vi "1L17_theC-T-en-Volts.vi"(5 "Temperature Units":u16(ring) caption="Unités de température" items=["Celsius", "Fahrenheit", "Kelvin", "Rankine"], 6 "ThermocoupleType":u16(ring)=2 caption="TypeThermocouple" items=["B", "E", "J", "K", "R", "S", "T", "N"], 7 "Temperature":sgl caption="Température" format="%0.6f") -> (3 "Thermocouple Voltage":sgl caption="Tension du thermocouple" format="%0.6f")   [LabVIEW 2010, in "lv_01.lvlib"]
doc: "Convertit une température en tension de thermocouple.\n\nNational Instruments a choisi des expressions polynomiales de thermocouple qui ne sont valides que pour des gammes de températures spécifiques (indiquées sur le diagramme du VI). Ces polynômes proviennent des tables NIST Monograph 175.\n\nPour utiliser une autre formule de conversion, vous pouvez éditer ce VI et entrer votre propre formule dans la boîte de calcul appropriée."
uses:
  lv_01.lvlib
panel:
  # "Convertit une température en une tension de thermocouple."
  # "National Instruments a sélectionné des expressions polynomiale de thermocouple qui ne sont valides que pour des gammes de températures particulières (données dans le diagramme du VI)  Ces polynômes proviennent des tables NIST Monograph 175.\n\nPour utiliser une autre formule de conversion, vous pouvez éditer ce VI et entrer votre propre formule dans la boîte de calcul appropriée."
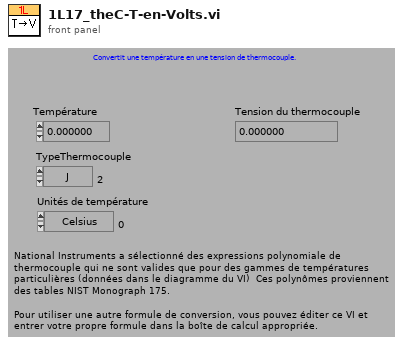
[diagram p1: front panel]
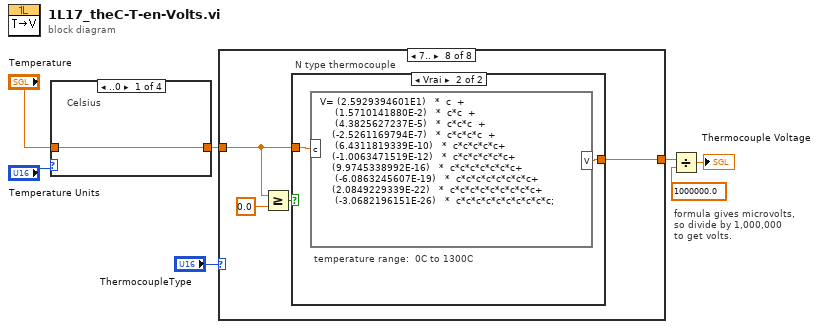
[diagram p0: block diagram]
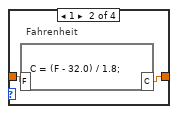
[diagram p2: hidden frame]
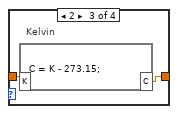
[diagram p3: hidden frame]
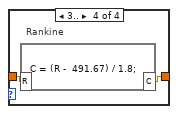
[diagram p4: hidden frame]
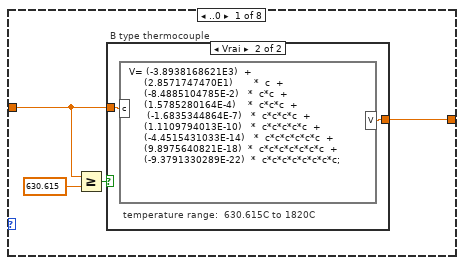
[diagram p5: hidden frame]
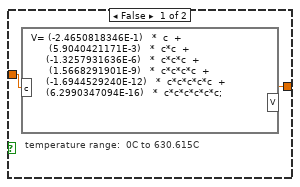
[diagram p6: hidden frame]
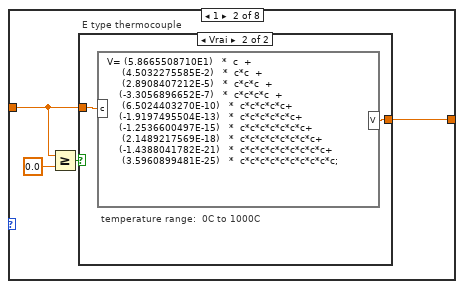
[diagram p7: hidden frame]
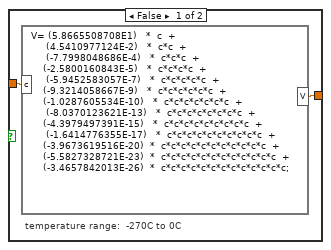
[diagram p8: hidden frame]
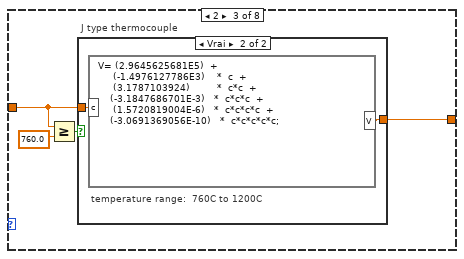
[diagram p9: hidden frame]
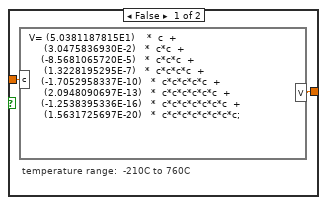
[diagram p10: hidden frame]
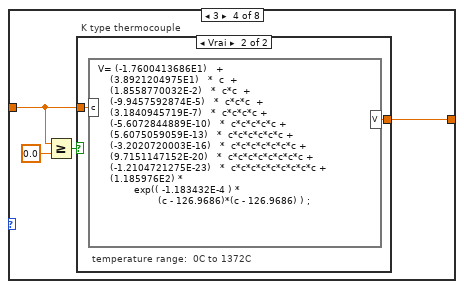
[diagram p11: hidden frame]
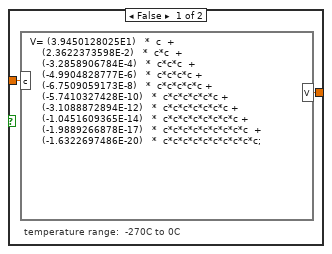
[diagram p12: hidden frame]
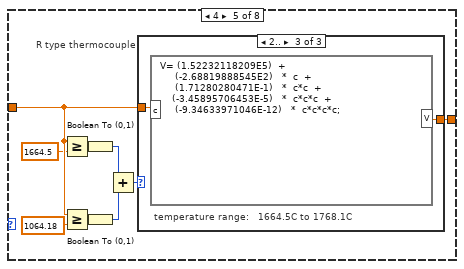
[diagram p13: hidden frame]
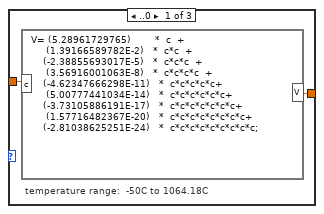
[diagram p14: hidden frame]
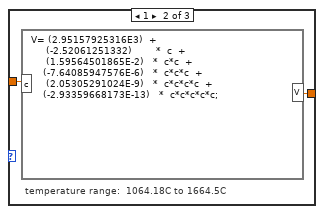
[diagram p15: hidden frame]
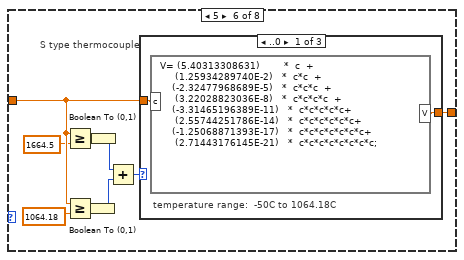
[diagram p16: hidden frame]
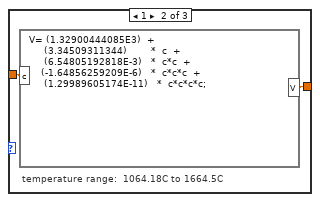
[diagram p17: hidden frame]
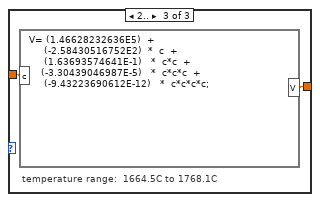
[diagram p18: hidden frame]
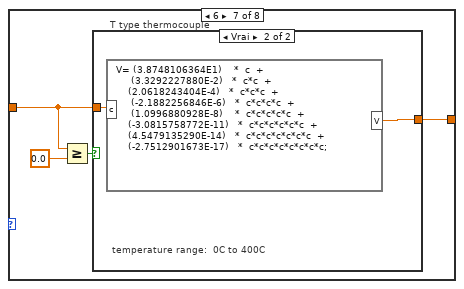
[diagram p19: hidden frame]
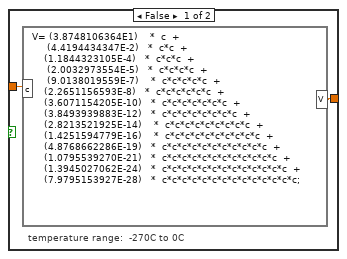
[diagram p20: hidden frame]
diagram:
  # "formula gives microvolts,\nso divide by 1,000,000\nto get volts."
  n1 = case shown="..0" "Temperature Units" {
    tunnel: "Temperature" -> [w8 w10 w12 w14]
    tunnel: [w8 w9 w11 w13] -> w6
    frame ..0 {
      # "Celsius"
    }
    frame 1 {
      # "Fahrenheit"
      n2 = formula code="C = (F - 32.0) / 1.8;"("F"=w10) -> ("C"=w9:dbl)
    }
    frame 2 {
      # "Kelvin"
      n3 = formula code="C = K - 273.15;"("K"=w12) -> ("C"=w11:dbl)
    }
    frame 3.. {
      # "Rankine"
      n4 = formula code="C = (R -  491.67) / 1.8;"("R"=w14) -> ("C"=w13:dbl)
    }
  }
  n5 = case shown="7.." "ThermocoupleType" {
    tunnel: [w15 w26 w34 w42 w55 w70 w80 w85] -> w3
    tunnel: w6 -> [w17 w24 w32 w40 w53 w68 w78 w86]
    frame ..0 {
      # "B type thermocouple"
      n6 = Greater Or Equal?(x=w17, y=630.615) -> (x >= y?=w18:bool)
      n7 = case shown="Vrai" w18 {
        tunnel: w17 -> [w19 w22]
        tunnel: [w20 w21] -> w15
        frame False {
          # "temperature range:  0C to 630.615C"
          n8 = formula code="V= (-2.4650818346E-1)   *  c  +\n      (5.9040421171E-3)   *  c*c  +\n     (-1.3257931636E-6)   *  c*c*c  +\n      (1.5668291901E-9)   *  c*c*c*c  +\n     (-1.6944529240E-12)   *  c*c*c*c*c  +\n     (6.2990347094E-16)   *  c*c*c*c*c*c;"("c"=w19) -> ("V"=w20:dbl)
        }
        frame True {
          # "temperature range:  630.615C to 1820C"
          n9 = formula code="V= (-3.8938168621E3)  +\n     (2.8571747470E1)       *  c  +\n     (-8.4885104785E-2)   *  c*c  +\n     (1.5785280164E-4)    *  c*c*c  +\n      (-1.6835344864E-7)   *  c*c*c*c  +\n     (1.1109794013E-10)   *  c*c*c*c*c  +\n     (-4.4515431033E-14)   *  c*c*c*c*c*c  +\n     (9.8975640821E-18)  *  c*c*c*c*c*c*c  +\n     (-9.3791330289E-22)  *  c*c*c*c*c*c*c*c;"("c"=w22) -> ("V"=w21:dbl)
        }
      }
    }
    frame 1 {
      # "E type thermocouple"
      n10 = Greater Or Equal?(x=w24, y=0.0) -> (x >= y?=w25:bool)
      n11 = case shown="Vrai" w25 {
        tunnel: w24 -> [w28 w30]
        tunnel: [w27 w29] -> w26
        frame False {
          # "temperature range:  -270C to 0C"
          n12 = formula code="V= (5.8665508708E1)   *  c  +\n     (4.5410977124E-2)   *  c*c  +\n     (-7.7998048686E-4)   *  c*c*c  +\n    (-2.5800160843E-5)   *  c*c*c*c  +\n     (-5.9452583057E-7)   *  c*c*c*c*c  +\n    (-9.3214058667E-9)   *  c*c*c*c*c*c  +\n    (-1.0287605534E-10)   *  c*c*c*c*c*c*c  +\n     (-8.0370123621E-13)   *  c*c*c*c*c*c*c*c  +\n    (-4.3979497391E-15)   *  c*c*c*c*c*c*c*c*c  +\n     (-1.6414776355E-17)   *  c*c*c*c*c*c*c*c*c*c  +\n    (-3.9673619516E-20)  *  c*c*c*c*c*c*c*c*c*c*c  +\n    (-5.5827328721E-23)  *  c*c*c*c*c*c*c*c*c*c*c*c  +\n    (-3.4657842013E-26)  *  c*c*c*c*c*c*c*c*c*c*c*c*c;"("c"=w28) -> ("V"=w27:dbl)
        }
        frame True {
          # "temperature range:  0C to 1000C"
          n13 = formula code="V= (5.8665508710E1)   *  c  +\n     (4.5032275585E-2)   *  c*c  +\n     (2.8908407212E-5)   *  c*c*c  +\n    (-3.3056896652E-7)   *  c*c*c*c  +\n     (6.5024403270E-10)   *  c*c*c*c*c+\n    (-1.9197495504E-13)   *  c*c*c*c*c*c+\n    (-1.2536600497E-15)   *  c*c*c*c*c*c*c+\n     (2.1489217569E-18)   *  c*c*c*c*c*c*c*c+\n    (-1.4388041782E-21)   *  c*c*c*c*c*c*c*c*c+\n     (3.5960899481E-25)   *  c*c*c*c*c*c*c*c*c*c;"("c"=w30) -> ("V"=w29:dbl)
        }
      }
    }
    frame 2 {
      # "J type thermocouple"
      n14 = Greater Or Equal?(x=w32, y=760.0) -> (x >= y?=w33:bool)
      n15 = case shown="Vrai" w33 {
        tunnel: [w36 w38] -> w34
        tunnel: w32 -> [w35 w37]
        frame False {
          # "temperature range:  -210C to 760C"
          n16 = formula code="V= (5.0381187815E1)    *  c  +\n     (3.0475836930E-2)   *  c*c  +\n    (-8.5681065720E-5)   *  c*c*c  +\n     (1.3228195295E-7)   *  c*c*c*c  +\n    (-1.7052958337E-10)   *  c*c*c*c*c  +\n     (2.0948090697E-13)   *  c*c*c*c*c*c  +\n    (-1.2538395336E-16)   *  c*c*c*c*c*c*c  +\n     (1.5631725697E-20)   *  c*c*c*c*c*c*c*c;"("c"=w35) -> ("V"=w36:dbl)
        }
        frame True {
          # "temperature range:  760C to 1200C"
          n17 = formula code="V= (2.9645625681E5)  +\n     (-1.4976127786E3)    *  c  +\n     (3.1787103924)         *  c*c  +\n    (-3.1847686701E-3)   *  c*c*c  +\n     (1.5720819004E-6)   *  c*c*c*c  +\n    (-3.0691369056E-10)   *  c*c*c*c*c;"("c"=w37) -> ("V"=w38:dbl)
        }
      }
    }
    frame 3 {
      # "K type thermocouple"
      n18 = Greater Or Equal?(x=w40, y=0.0) -> (x >= y?=w41:bool)
      n19 = case shown="Vrai" w41 {
        tunnel: w40 -> [w44 w46]
        tunnel: [w43 w45] -> w42
        frame False {
          # "temperature range:  -270C to 0C"
          n20 = formula code="V= (3.9450128025E1)   *  c  +\n    (2.3622373598E-2)   *  c*c  +\n    (-3.2858906784E-4)   *  c*c*c  +\n    (-4.9904828777E-6)   *  c*c*c*c +\n    (-6.7509059173E-8)   *  c*c*c*c*c +\n    (-5.7410327428E-10)   *  c*c*c*c*c*c +\n    (-3.1088872894E-12)   *  c*c*c*c*c*c*c +\n    (-1.0451609365E-14)   *  c*c*c*c*c*c*c*c +\n    (-1.9889266878E-17)   *  c*c*c*c*c*c*c*c*c  +\n    (-1.6322697486E-20)   *  c*c*c*c*c*c*c*c*c*c;"("c"=w44) -> ("V"=w43:dbl)
        }
        frame True {
          # "temperature range:  0C to 1372C"
          n21 = formula code="V= (-1.7600413686E1)   +\n    (3.8921204975E1)   *  c  +\n    (1.8558770032E-2)   *  c*c  +\n    (-9.9457592874E-5)   *  c*c*c  +\n    (3.1840945719E-7)   *  c*c*c*c +\n    (-5.6072844889E-10)   *  c*c*c*c*c +\n    (5.6075059059E-13)   *  c*c*c*c*c*c +\n    (-3.2020720003E-16)   *  c*c*c*c*c*c*c +\n    (9.7151147152E-20)   *  c*c*c*c*c*c*c*c +\n    (-1.2104721275E-23)   *  c*c*c*c*c*c*c*c*c +\n    (1.185976E2) * \n            exp(( -1.183432E-4 ) * \n                    (c - 126.9686)*(c - 126.9686) ) ;"("c"=w46) -> ("V"=w45:dbl)
        }
      }
    }
    frame 4 {
      # "R type thermocouple"
      n22 = Greater Or Equal?(x=w53, y=1664.5) -> (x >= y?=w50:bool)
      n23 = Greater Or Equal?(x=w53, y=1064.18) -> (x >= y?=w49:bool)
      n24 = Boolean To (0,1)(Boolean=w50) -> (0, 1=w47:i16)
      n25 = Boolean To (0,1)(Boolean=w49) -> (0, 1=w48:i16)
      n26 = Add(x=w47, y=w48) -> (x+y=w54:i16)
      n27 = case shown="2.." w54 {
        tunnel: w53 -> [w57 w59 w61]
        tunnel: [w56 w58 w60] -> w55
        frame ..0 {
          # "temperature range:  -50C to 1064.18C"
          n28 = formula code="V= (5.28961729765)        *  c  +\n     (1.39166589782E-2)   *  c*c  +\n    (-2.38855693017E-5)   *  c*c*c  +\n     (3.56916001063E-8)   *  c*c*c*c  +\n    (-4.62347666298E-11)   *  c*c*c*c*c+\n     (5.00777441034E-14)   *  c*c*c*c*c*c+\n    (-3.73105886191E-17)   *  c*c*c*c*c*c*c+\n     (1.57716482367E-20)   *  c*c*c*c*c*c*c*c+\n    (-2.81038625251E-24)   *  c*c*c*c*c*c*c*c*c;"("c"=w57) -> ("V"=w56:dbl)
        }
        frame 1 {
          # "temperature range:  1064.18C to 1664.5C"
          n29 = formula code="V= (2.95157925316E3)  +\n     (-2.52061251332)        *  c  +\n     (1.59564501865E-2)   *  c*c  +\n    (-7.64085947576E-6)   *  c*c*c  +\n     (2.05305291024E-9)   *  c*c*c*c  +\n    (-2.93359668173E-13)   *  c*c*c*c*c;"("c"=w59) -> ("V"=w58:dbl)
        }
        frame 2.. {
          # "temperature range:   1664.5C to 1768.1C"
          n30 = formula code="V= (1.52232118209E5)  +\n     (-2.68819888545E2)   *  c  +\n     (1.71280280471E-1)   *  c*c  +\n    (-3.45895706453E-5)   *  c*c*c  +\n     (-9.34633971046E-12)   *  c*c*c*c;"("c"=w61) -> ("V"=w60:dbl)
        }
      }
    }
    frame 5 {
      # "S type thermocouple"
      n31 = Greater Or Equal?(x=w68, y=1664.5) -> (x >= y?=w65:bool)
      n32 = Greater Or Equal?(x=w68, y=1064.18) -> (x >= y?=w64:bool)
      n33 = Boolean To (0,1)(Boolean=w64) -> (0, 1=w63:i16)
      n34 = Boolean To (0,1)(Boolean=w65) -> (0, 1=w62:i16)
      n35 = Add(x=w62, y=w63) -> (x+y=w69:i16)
      n36 = case shown="..0" w69 {
        tunnel: w68 -> [w72 w74 w76]
        tunnel: [w71 w73 w75] -> w70
        frame ..0 {
          # "temperature range:  -50C to 1064.18C"
          n37 = formula code="V= (5.40313308631)        *  c  +\n     (1.25934289740E-2)   *  c*c  +\n    (-2.32477968689E-5)   *  c*c*c  +\n     (3.22028823036E-8)   *  c*c*c*c  +\n    (-3.31465196389E-11)   *  c*c*c*c*c+\n     (2.55744251786E-14)   *  c*c*c*c*c*c+\n    (-1.25068871393E-17)   *  c*c*c*c*c*c*c+\n     (2.71443176145E-21)   *  c*c*c*c*c*c*c*c;"("c"=w72) -> ("V"=w71:dbl)
        }
        frame 1 {
          # "temperature range:  1064.18C to 1664.5C"
          n38 = formula code="V= (1.32900444085E3)  +\n     (3.34509311344)        *  c  +\n     (6.54805192818E-3)   *  c*c  +\n    (-1.64856259209E-6)   *  c*c*c  +\n     (1.29989605174E-11)   *  c*c*c*c;"("c"=w74) -> ("V"=w73:dbl)
        }
        frame 2.. {
          # "temperature range:  1664.5C to 1768.1C"
          n39 = formula code="V= (1.46628232636E5)  +\n     (-2.58430516752E2)  *  c  +\n     (1.63693574641E-1)   *  c*c  +\n    (-3.30439046987E-5)   *  c*c*c  +\n     (-9.43223690612E-12)   *  c*c*c*c;"("c"=w76) -> ("V"=w75:dbl)
        }
      }
    }
    frame 6 {
      # "T type thermocouple"
      n40 = Greater Or Equal?(x=w78, y=0.0) -> (x >= y?=w79:bool)
      n41 = case shown="Vrai" w79 {
        tunnel: w78 -> [w82 w84]
        tunnel: [w81 w83] -> w80
        frame False {
          # "temperature range:  -270C to 0C"
          n42 = formula code="V= (3.8748106364E1)    *  c  +\n     (4.4194434347E-2)   *  c*c  +\n    (1.1844323105E-4)   *  c*c*c  +\n     (2.0032973554E-5)   *  c*c*c*c  +\n     (9.0138019559E-7)    *  c*c*c*c*c  +\n    (2.2651156593E-8)   *  c*c*c*c*c*c  +\n    (3.6071154205E-10)   *  c*c*c*c*c*c*c  +\n    (3.8493939883E-12)   *  c*c*c*c*c*c*c*c  +\n    (2.8213521925E-14)    *  c*c*c*c*c*c*c*c*c  +\n    (1.4251594779E-16)    *  c*c*c*c*c*c*c*c*c*c  +\n    (4.8768662286E-19)   *  c*c*c*c*c*c*c*c*c*c*c  +\n    (1.0795539270E-21)   *  c*c*c*c*c*c*c*c*c*c*c*c  +\n    (1.3945027062E-24)   *  c*c*c*c*c*c*c*c*c*c*c*c*c  +\n    (7.9795153927E-28)   *  c*c*c*c*c*c*c*c*c*c*c*c*c*c;"("c"=w82) -> ("V"=w81:dbl)
        }
        frame True {
          # "temperature range:  0C to 400C"
          n43 = formula code="V= (3.8748106364E1)    *  c  +\n     (3.3292227880E-2)   *  c*c  +\n    (2.0618243404E-4)   *  c*c*c  +\n     (-2.1882256846E-6)   *  c*c*c*c  +\n     (1.0996880928E-8)    *  c*c*c*c*c  +\n    (-3.0815758772E-11)   *  c*c*c*c*c*c  +\n    (4.5479135290E-14)   *  c*c*c*c*c*c*c  +\n    (-2.7512901673E-17)   *  c*c*c*c*c*c*c*c;"("c"=w84) -> ("V"=w83:dbl)
        }
      }
    }
    frame 7.. {
      # "N type thermocouple"
      n44 = Greater Or Equal?(x=w86, y=0.0) -> (x >= y?=w88:bool)
      n45 = case shown="Vrai" w88 {
        tunnel: w86 -> [w90 w92]
        tunnel: [w89 w91] -> w85
        frame False {
          # "temperature range:  -270C to 0C"
          n46 = formula code="V= (2.6159105962E1)   *  c  +\n     (1.0957484228E-2)   *  c*c  +\n     (-9.3841111554E-5)   *  c*c*c  +\n    (-4.6412039759E-8)   *  c*c*c*c  +\n     (-2.6303357716E-9)   *  c*c*c*c*c  +\n    (-2.2653438003E-11)   *  c*c*c*c*c*c  +\n    (-7.6089300791E-14)   *  c*c*c*c*c*c*c  +\n     (-9.3419667835E-17)   *  c*c*c*c*c*c*c*c;"("c"=w90) -> ("V"=w89:dbl)
        }
        frame True {
          # "temperature range:  0C to 1300C"
          n47 = formula code="V= (2.5929394601E1)   *  c  +\n     (1.5710141880E-2)   *  c*c  +\n     (4.3825627237E-5)   *  c*c*c  +\n    (-2.5261169794E-7)   *  c*c*c*c  +\n     (6.4311819339E-10)   *  c*c*c*c*c+\n    (-1.0063471519E-12)   *  c*c*c*c*c*c+\n    (9.9745338992E-16)   *  c*c*c*c*c*c*c+\n     (-6.0863245607E-19)   *  c*c*c*c*c*c*c*c+\n    (2.0849229339E-22)   *  c*c*c*c*c*c*c*c*c+\n     (-3.0682196151E-26)   *  c*c*c*c*c*c*c*c*c*c;"("c"=w92) -> ("V"=w91:dbl)
        }
      }
    }
  }
  n48 = Divide(x=w3, y=1000000.0) -> (x/y=→"Thermocouple Voltage":dbl)
